vi "Init.vi"(6 "Compression?":bool, 7 "Prepend Result Name":bool, 8 "error in (no error)":errorcluster, 9 "SA Pin":string, 10 "Measurement Name":string, 11 "Standard":string) -> (0 "error out":errorcluster, 3 "Servo Gain out":refnum<class "Servo Gain.lvclass">)   [LabVIEW 2016, in "SeqAuto Evaluations.lvlib" / "Servo Gain.lvclass"]
uses:
  Servo Gain.lvclass
  C:/Sequence Automation/Plugins/SeqAuto IEvaluation.lvlibp/SeqAuto IEvaluation.lvclass
  Servo Gain.lvclass/Servo Gain.ctl
  Plugins/SeqAuto IEvaluation.lvlibp/Write Measurement Name.vi
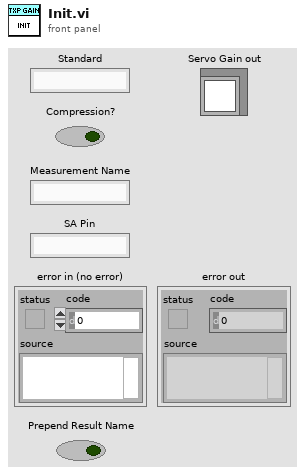
[diagram p1: front panel]
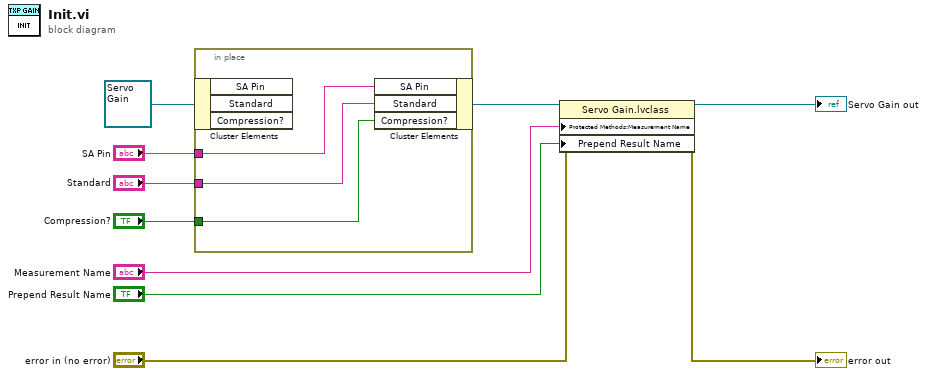
[diagram p0: block diagram]
diagram:
  n1 = in-place {
    in-place-border: "SA Pin" -> [w13]
    in-place-border: "Standard" -> [w12]
    in-place-border: "Compression?" -> [w11]
    n2 = in-place-cluster #1(refnum<class "Servo Gain.lvclass"> refnum ("Servo Gain in")) -> ()  [unwired: 3 out]
    n3 = in-place-cluster #1("SA Pin"=w13, "Standard"=w12, "Compression?"=w11) -> (w6:refnum<class "Servo Gain.lvclass">)
  }
  n4 = property class="Servo Gain.lvclass"(reference=w6, error in="error in (no error)", "Protected Methods:Measurement Name"="Measurement Name", "Prepend Result Name"="Prepend Result Name") -> (reference out=→"Servo Gain out":refnum<class "Servo Gain.lvclass">, error out=→"error out":errorcluster)
